vi "_Parse SEM Extreme Result.vi"(8 "error in (no error)":errorcluster, 10 "Input String":string, 11 "VISA resource name":refnum<visa-resource-name>) -> (0 "error out":errorcluster, 1 "SEM Extreme Results":T1 {"TX Power Max" format="%^.3e"; "TX Power Min" format="%^.3e"; "Occupied Bandwidth" format="%^.3e"}, 2 "Reliability":i32, 3 "VISA resource name out":refnum<visa-resource-name>, 5 "Out Of Tolerance":i32)   [LabVIEW 2020, in "Rohde&Schwarz CMWXP NR FR1 Measurement.lvlib"]
uses:
  <instrlib>/Rohde&Schwarz CMWXP NR FR1 Measurement/Rohde&Schwarz CMWXP NR FR1 Measurement.lvlib
  <instrlib>/Rohde&Schwarz CMWXP NR FR1 Measurement/Private/rsidr_core.llb/rsidr_core.lvlib
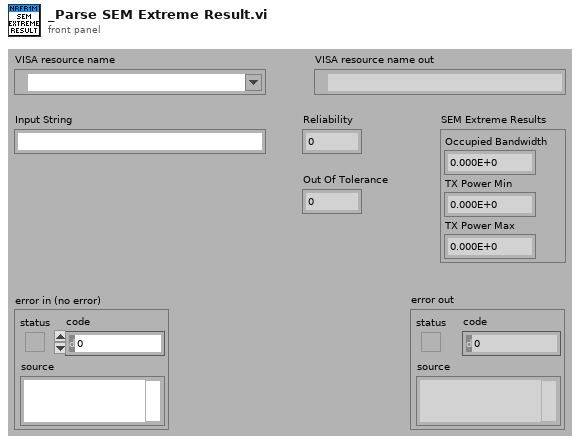
[diagram p1: front panel]
types:
  T1 = cluster{"Occupied Bandwidth":dbl, "TX Power Min":dbl, "TX Power Max":dbl}
  T2 = cluster{"double value out":dbl, "double value out":dbl, "double value out":dbl}
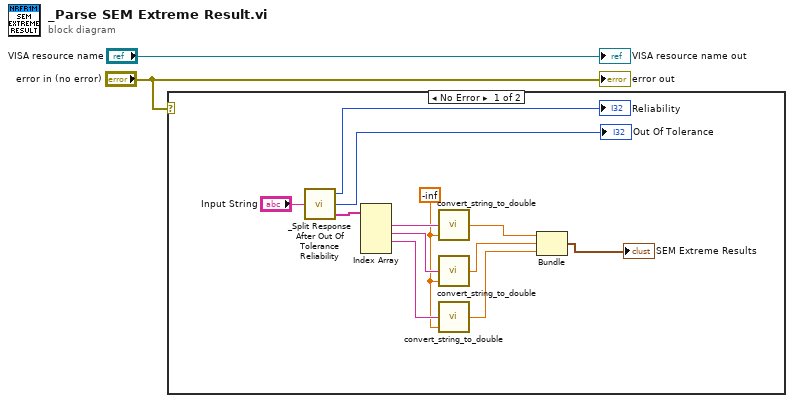
[diagram p0: block diagram]
diagram:
  n1 = case shown="No Error" "error in (no error)" {
    frame No Error {
      w5 = -inf
      n2 = call <instrlib>:"_Split Response After Out Of Tolerance Reliability.vi"("Input String"="Input String") -> ("Reliability out"=→"Reliability":i32, "Out Of Tolerance"=→"Out Of Tolerance":i32, "Response out"=w9:string[])
      n3 = Index Array(array=w9) -> (element #1=w8:string, element #2=w7:string, element #3=w6:string)  [unwired: 4 in, 1 out]
      n4 = call <instrlib>:"convert_string_to_double.vi"("default (0)"=w5, "String in"=w8) -> ("double value out"=w14:dbl)  [unwired: 3 in]
      n5 = call <instrlib>:"convert_string_to_double.vi"("default (0)"=w5, "String in"=w7) -> ("double value out"=w13:dbl)  [unwired: 3 in]
      n6 = call <instrlib>:"convert_string_to_double.vi"("default (0)"=w5, "String in"=w6) -> ("double value out"=w12:dbl)  [unwired: 3 in]
      n7 = Bundle("double value out"=w14, "double value out"=w13, "double value out"=w12) -> (→"SEM Extreme Results":T2)  [unwired: 1 in]
    }
    frame Error {
    }
  }
  "error out" <- "error in (no error)"
  "VISA resource name out" <- "VISA resource name"
